vi "Write Menu Selection.vi"(8 "error in (no error)":errorcluster, 10 "Menu Selection":refnum<user-event>, 11 "Table Manager in":refnum<class "Table Manager.lvclass">) -> (0 "error out":errorcluster, 3 "Table Manager out":refnum<class "Table Manager.lvclass">)   [LabVIEW 2013, in "Table Manager.lvlib" / "Table Manager.lvclass"]
uses:
  Table Manager.lvclass
  Menu Select.ctl
  Table Manager.lvclass/Table Manager.ctl
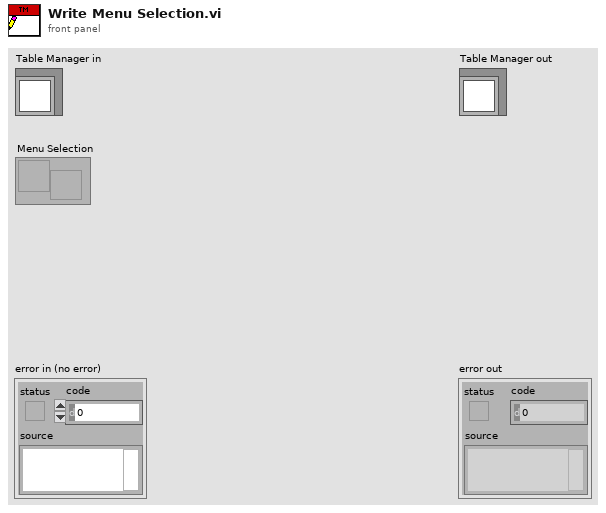
[diagram p1: front panel]
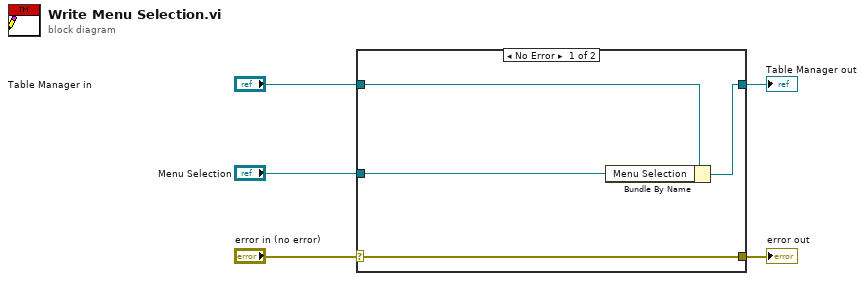
[diagram p0: block diagram]
diagram:
  n1 = case shown="No Error" "error in (no error)" {
    selector: "error in (no error)" -> [w9 w10]
    tunnel: [w9 w10] -> w4
    tunnel: [w7 w11] -> w2
    tunnel: "Table Manager in" -> [w8 w11]
    tunnel: "Menu Selection" -> [w6 _]
    frame No Error {
      n2 = Bundle By Name(cluster=w8, "Menu Selection"=w6) -> (w7:refnum<class "Table Manager.lvclass">)
    }
    frame Error {
    }
  }
  "error out" <- w4
  "Table Manager out" <- w2
